vi "Analog Out Region.vi"(6 "aout limit":T1={"ALimUpC"=10.5, "ALimUpL"=10.0, "ALimLoC"=-10.0, "ALimLoL"=-10.0}, 8 "aout point":T3, 9 "aout bounds":T2={"ABndUpC"=10.0, "ABndUpL"=10.0, "ABndLoC"=-10.0, "ABndLoL"=-10.0}, 10 "dev point":T5={"dev point cap"=100.0, "dev point loss"=0.0}, 11 "dev bounds":T4) -> (0 "Loss Analog Output":cluster{cluster{dbl, dbl}[]}[](graph), 3 "Capacitance Analog Output":cluster{cluster{dbl, dbl}[]}[](graph))   [LabVIEW 2024, in "Andeen-Hagerling 2700A.lvlib"]
doc: "Generates graphs representing capacitance and loss analog output."
uses:
  Andeen-Hagerling 2700A.lvlib
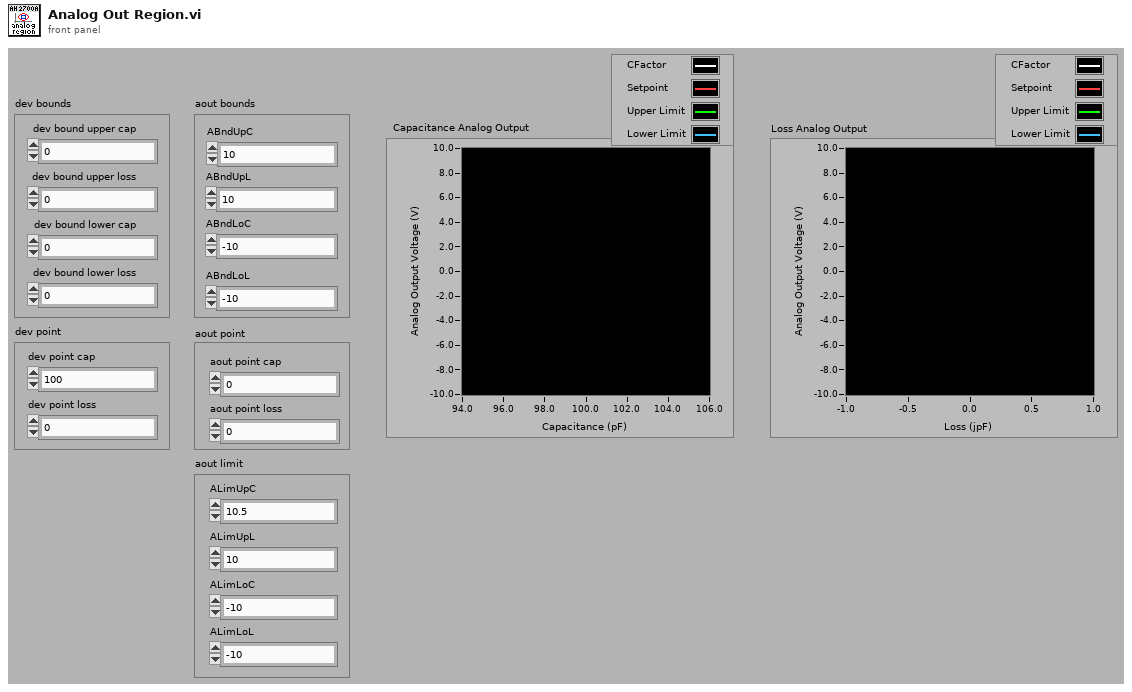
[diagram p1: front panel]
types:
  T1 = cluster{"ALimUpC":dbl, "ALimUpL":dbl, "ALimLoC":dbl, "ALimLoL":dbl}
  T2 = cluster{"ABndUpC":dbl, "ABndUpL":dbl, "ABndLoC":dbl, "ABndLoL":dbl}
  T3 = cluster{"aout point cap":dbl, "aout point loss":dbl}
  T4 = cluster{"dev bound upper cap":dbl, "dev bound upper loss":dbl, "dev bound lower cap":dbl, "dev bound lower loss":dbl}
  T5 = cluster{"dev point cap":dbl, "dev point loss":dbl}
  T6 = cluster{"dev bound lower cap":dbl, "ABndLoC":dbl}
  T7 = cluster{"dev bound upper cap":dbl, "ABndUpC":dbl}
  T8 = cluster{"dev point cap":dbl, "aout point cap":dbl}
  T9 = cluster{"dev bound lower loss":dbl, "ABndLoL":dbl}
  T10 = cluster{"dev bound upper loss":dbl, "ABndUpL":dbl}
  T11 = cluster{"dev point loss":dbl, "aout point loss":dbl}
  T12 = cluster{"dev bound lower cap":dbl, "ALimUpC":dbl}
  T13 = cluster{"dev bound upper cap":dbl, "ALimUpC":dbl}
  T14 = cluster{"dev bound lower cap":dbl, "ALimLoC":dbl}
  T15 = cluster{"dev bound upper cap":dbl, "ALimLoC":dbl}
  T16 = cluster{"dev bound lower loss":dbl, "ALimUpL":dbl}
  T17 = cluster{"dev bound upper loss":dbl, "ALimUpL":dbl}
  T18 = cluster{"dev bound lower loss":dbl, "ALimLoL":dbl}
  T19 = cluster{"dev bound upper loss":dbl, "ALimLoL":dbl}
  T20 = cluster{"dev bound upper cap":dbl, "ABndUpC":dbl}[]
  T21 = cluster{"dev point cap":dbl, "aout point cap":dbl}[]
  T22 = cluster{"dev bound upper loss":dbl, "ABndUpL":dbl}[]
  T23 = cluster{"dev point loss":dbl, "aout point loss":dbl}[]
  T24 = cluster{"dev bound upper cap":dbl, "ALimUpC":dbl}[]
  T25 = cluster{"dev bound upper cap":dbl, "ALimLoC":dbl}[]
  T26 = cluster{"dev bound upper loss":dbl, "ALimUpL":dbl}[]
  T27 = cluster{"dev bound upper loss":dbl, "ALimLoL":dbl}[]
  T28 = cluster{cluster{"dev bound upper cap":dbl, "ABndUpC":dbl}[]}
  T29 = cluster{cluster{"dev point cap":dbl, "aout point cap":dbl}[]}
  T30 = cluster{cluster{"dev bound upper cap":dbl, "ALimUpC":dbl}[]}
  T31 = cluster{cluster{"dev bound upper cap":dbl, "ALimLoC":dbl}[]}
  T32 = cluster{cluster{"dev bound upper loss":dbl, "ABndUpL":dbl}[]}
  T33 = cluster{cluster{"dev point loss":dbl, "aout point loss":dbl}[]}
  T34 = cluster{cluster{"dev bound upper loss":dbl, "ALimUpL":dbl}[]}
  T35 = cluster{cluster{"dev bound upper loss":dbl, "ALimLoL":dbl}[]}
  T36 = cluster{cluster{"dev bound upper cap":dbl, "ALimLoC":dbl}[]}[]
  T37 = cluster{cluster{"dev bound upper loss":dbl, "ALimLoL":dbl}[]}[]
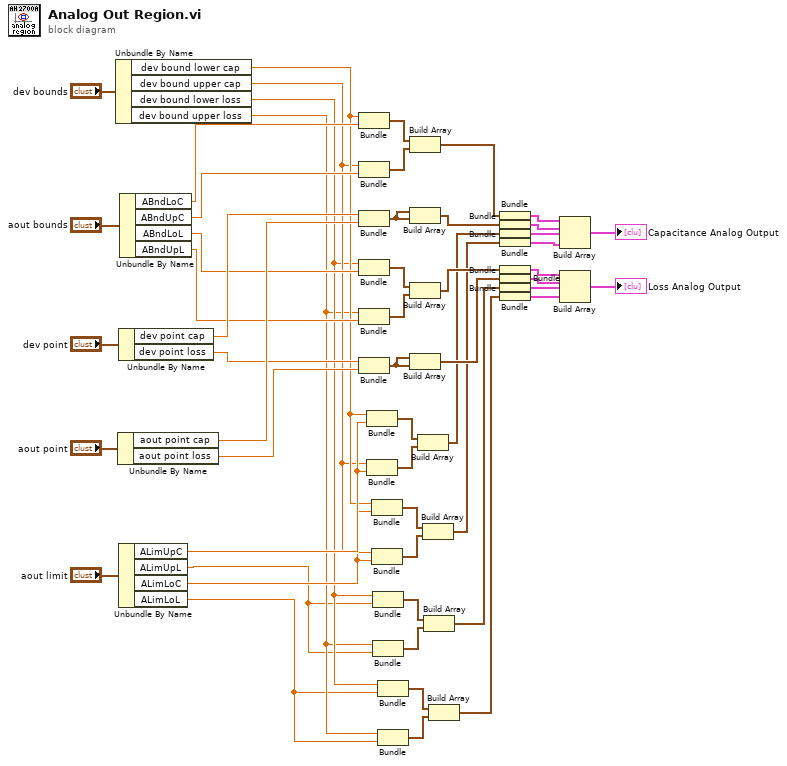
[diagram p0: block diagram]
diagram:
  n1 = Unbundle By Name("dev bounds") -> ("dev bound lower cap"=w17:dbl, "dev bound upper cap"=w16:dbl, "dev bound lower loss"=w8:dbl, "dev bound upper loss"=w7:dbl)
  n2 = Unbundle By Name("aout point") -> ("aout point cap"=w45:dbl, "aout point loss"=w32:dbl)
  n3 = Unbundle By Name("dev point") -> ("dev point cap"=w46:dbl, "dev point loss"=w33:dbl)
  n4 = Unbundle By Name("aout limit") -> ("ALimUpC"=w22:dbl, "ALimUpL"=w6:dbl, "ALimLoC"=w15:dbl, "ALimLoL"=w5:dbl)
  n5 = Unbundle By Name("aout bounds") -> ("ABndLoC"=w50:dbl, "ABndUpC"=w49:dbl, "ABndLoL"=w35:dbl, "ABndUpL"=w34:dbl)
  n6 = Bundle("dev bound lower cap"=w17, "ABndLoC"=w50) -> (w44:T6)  [unwired: 1 in]
  n7 = Bundle("dev bound upper cap"=w16, "ABndUpC"=w49) -> (w43:T7)  [unwired: 1 in]
  n8 = Bundle("dev point cap"=w46, "aout point cap"=w45) -> (w38:T8)  [unwired: 1 in]
  n9 = Bundle("dev bound lower loss"=w8, "ABndLoL"=w35) -> (w37:T9)  [unwired: 1 in]
  n10 = Bundle("dev bound upper loss"=w7, "ABndUpL"=w34) -> (w36:T10)  [unwired: 1 in]
  n11 = Bundle("dev point loss"=w33, "aout point loss"=w32) -> (w31:T11)  [unwired: 1 in]
  n12 = Bundle("dev bound lower cap"=w17, "ALimUpC"=w22) -> (w24:T12)  [unwired: 1 in]
  n13 = Bundle("dev bound upper cap"=w16, "ALimUpC"=w22) -> (w23:T13)  [unwired: 1 in]
  n14 = Bundle("dev bound lower cap"=w17, "ALimLoC"=w15) -> (w19:T14)  [unwired: 1 in]
  n15 = Bundle("dev bound upper cap"=w16, "ALimLoC"=w15) -> (w18:T15)  [unwired: 1 in]
  n16 = Bundle("dev bound lower loss"=w8, "ALimUpL"=w6) -> (w12:T16)  [unwired: 1 in]
  n17 = Bundle("dev bound upper loss"=w7, "ALimUpL"=w6) -> (w11:T17)  [unwired: 1 in]
  n18 = Bundle("dev bound lower loss"=w8, "ALimLoL"=w5) -> (w10:T18)  [unwired: 1 in]
  n19 = Bundle("dev bound upper loss"=w7, "ALimLoL"=w5) -> (w9:T19)  [unwired: 1 in]
  n20 = Build Array(w44, w43) -> (w42:T20)
  n21 = Build Array(w38, w38) -> (w39:T21)
  n22 = Build Array(w37, w36) -> (w28:T22)
  n23 = Build Array(w31, w31) -> (w27:T23)
  n24 = Build Array(w24, w23) -> (w21:T24)
  n25 = Build Array(w19, w18) -> (w14:T25)
  n26 = Build Array(w12, w11) -> (w4:T26)
  n27 = Build Array(w10, w9) -> (w3:T27)
  n28 = Bundle(w42) -> (w41:T28)  [unwired: 1 in]
  n29 = Bundle(w39) -> (w40:T29)  [unwired: 1 in]
  n30 = Bundle(w21) -> (w20:T30)  [unwired: 1 in]
  n31 = Bundle(w14) -> (w13:T31)  [unwired: 1 in]
  n32 = Bundle(w28) -> (w30:T32)  [unwired: 1 in]
  n33 = Bundle(w27) -> (w29:T33)  [unwired: 1 in]
  n34 = Bundle(w4) -> (w2:T34)  [unwired: 1 in]
  n35 = Bundle(w3) -> (w1:T35)  [unwired: 1 in]
  n36 = Build Array(w41, w40, w20, w13) -> (→"Capacitance Analog Output":T36)
  n37 = Build Array(w30, w29, w2, w1) -> (→"Loss Analog Output":T37)
